vi "GUI TWM setup.vi"(0 "Common properties":T1={"Measurement status ref"=refnum, "TWM Status ref"=refnum, "Abort ref"=refnum, "Skip waiting ref"=refnum, "GNU Octave path"=path "C:/Program Files/GNU Octave/Octave-6.2.0/mingw64/bin", "TWM+QWTB path"=path "C:/Users/labina/Desktop/TWM-1.8.7.0-full/octprog", "lvlib path"=path "D:/martin/WAC/WACsw - github/control_software/Filter function meter/external libraries/GOLPI 0.7.3.1 source distribution LV 20.0 32 bit/lv_proc.dll", "TWM pipe"="\\\\.\\pipe\\TWM:server", "PJVS status ref"=refnum, "WAC path"=path ""}) -> (7 "Common properties out":T1={"Measurement status ref"=refnum, "TWM Status ref"=refnum, "Abort ref"=refnum, "Skip waiting ref"=refnum, "GNU Octave path"=path "C:/Program Files/GNU Octave/Octave-6.2.0/mingw64/bin", "TWM+QWTB path"=path "C:/Users/labina/Desktop/TWM-1.8.7.0-full/octprog", "lvlib path"=path "D:/martin/WAC/WACsw - github/control_software/Filter function meter/external libraries/GOLPI 0.7.3.1 source distribution LV 20.0 32 bit/lv_proc.dll", "TWM pipe"="\\\\.\\pipe\\TWM:server", "PJVS status ref"=refnum, "WAC path"=path ""})   [LabVIEW 2020]
doc: "GUI to set up connection to the sampling sotware TWM and to set up paths to calculation software GNU Octave."
uses:
  Utilities/Type definitions/Common properties.ctl
  <vilib>/Utility/error.llb/DialogType.ctl
  <vilib>/Utility/error.llb/Error Cluster From Error Code.vi
  <vilib>/ErrorRing/Error Ring.xnode
  external libraries/varilib/varilib.lvlib
  external libraries/TWM-1.8.7.0-client/TWM Client.lvlib
panel:
  in  "start octave":bool
  out "twm_qwtb_not_valid":string="not valid!"
  out "octave_not_valid":string="not valid!"
  in  "TWM+QWTB path":path=path "C:/Users/labina/Desktop/TWM-1.8.7.0-full/octprog"
  in  "GNU Octave path":path=path "C:/Program Files/GNU Octave/Octave-6.2.0/mingw64/bin"
  in  "TWM pipe":string="\\\\.\\pipe\\TWM:server"
  out "gui_elements":refnum<vi>[](array[refnum])
  out "Status":string
  in  "save_and_quit":bool
  in  "test TWM":bool
  in  "cancel":bool
  # "This software changes following properties\nin the TWM automatically before running \na measurement:\n1, Sampling rate (TWM->Setup Measurement)\n2, Samples count (TWM->Setup Measurement)\n3, Records count (TWM->Setup Measurement)\n4, Sub-records count (TWM->Setup Measurement)\n5, Trigger (mode, source, level, coupling\n                                     (TWM->Setup Measurment)\n6, Measurement name (TWM->Setup Measurement)\n7, Processing setup"
  # "You must set following in TWM\nby yourself:\n1, Octave/Matlab\n2, Digitizer"
  # "GNU Octave for calculation of results or recalculation of sampled data."
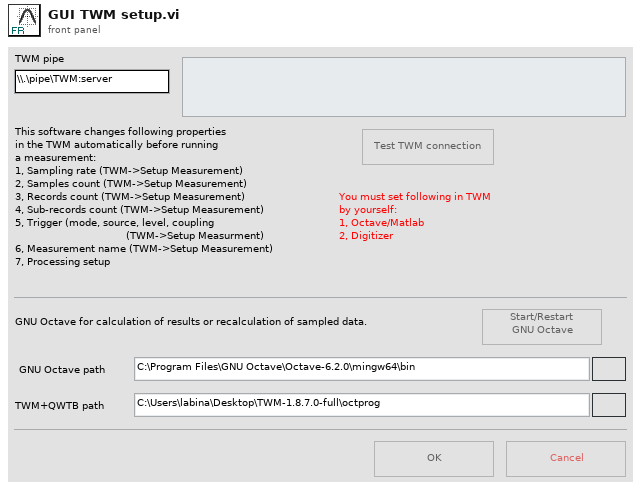
[diagram p1: front panel]
types:
  T1 = typedef "Common properties.ctl" = cluster{"Measurement status ref":refnum<vi>, "TWM Status ref":refnum<vi>, "Abort ref":refnum<vi>, "Skip waiting ref":refnum<vi>, "GNU Octave path":path, "TWM+QWTB path":path, "lvlib path":path, "TWM pipe":string, "PJVS status ref":refnum<vi>, "WAC path":path}
  T2 = typedef "DialogType.ctl" = u16
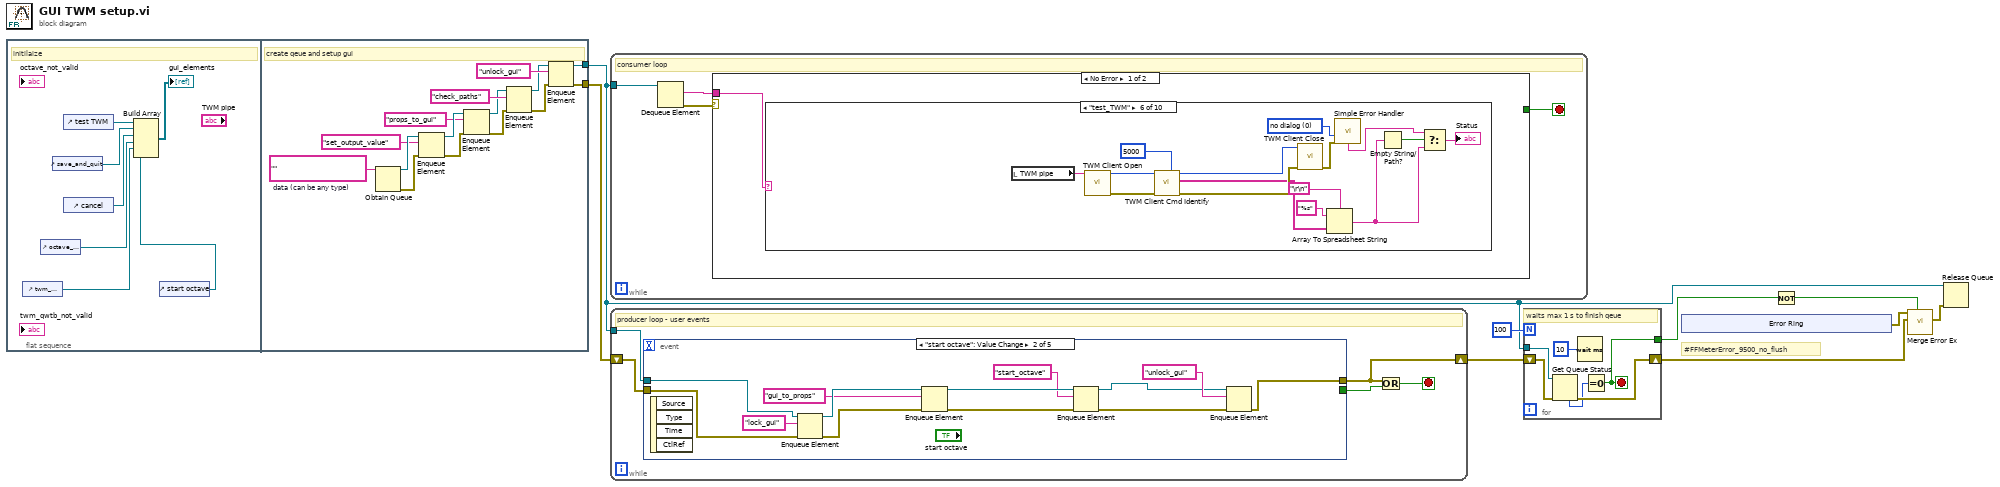
[diagram p0: block diagram]
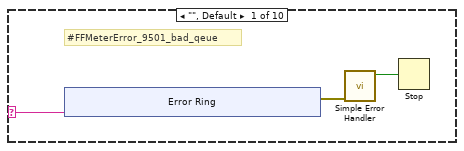
[diagram p2: hidden frame]
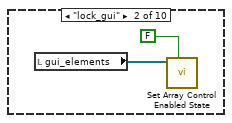
[diagram p3: hidden frame]
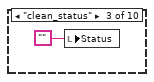
[diagram p4: hidden frame]
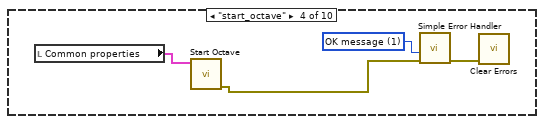
[diagram p5: hidden frame]
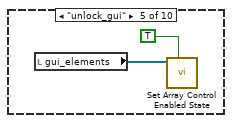
[diagram p6: hidden frame]
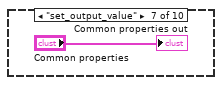
[diagram p7: hidden frame]
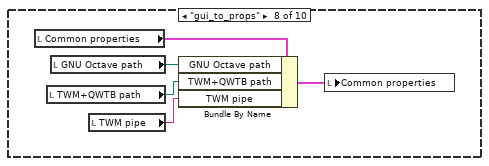
[diagram p8: hidden frame]
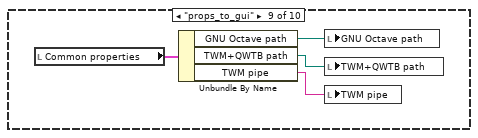
[diagram p9: hidden frame]
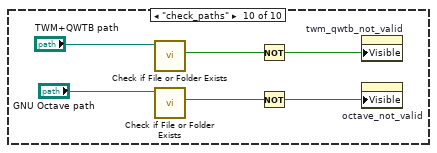
[diagram p10: hidden frame]
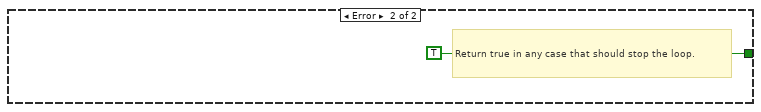
[diagram p11: hidden frame]
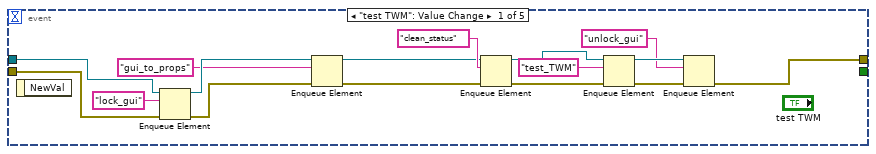
[diagram p12: hidden frame]
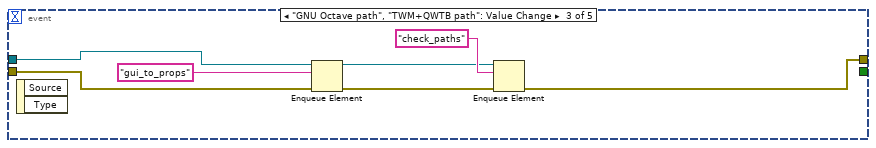
[diagram p13: hidden frame]
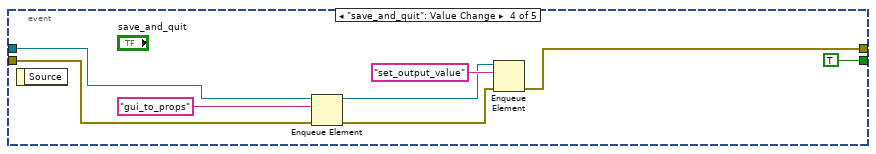
[diagram p14: hidden frame]
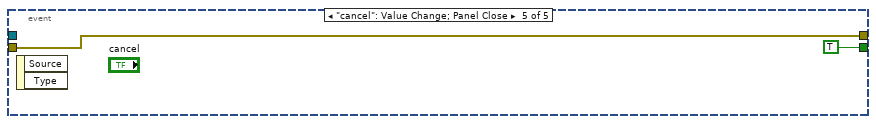
[diagram p15: hidden frame]
diagram:
  # "#FFMeterError_9500_no_flush"
  n1 = flat-sequence {
    tunnel: [w27] -> w2
    tunnel: [w25] -> w1
    frame #0 {
      # "initilaize"
      n2 = control-ref of="twm_qwtb_not_valid"() -> (w11:refnum<vi>)
      n3 = control-ref of="octave_not_valid"() -> (w12:refnum<vi>)
      n4 = control-ref of="save_and_quit"() -> (w15:refnum<vi>)
      n5 = control-ref of="test TWM"() -> (w16:refnum<vi>)
      n6 = control-ref of="cancel"() -> (w14:refnum<vi>)
      n7 = control-ref of="start octave"() -> (w10:refnum<vi>)
      n8 = Build Array(w16, w15, w14, w12, w11, w10) -> (→"gui_elements":refnum<vi>[])
    }
    frame #1 {
      w26 = ""  # data (can be any type)
      # "create qeue and setup gui"
      n9 = Obtain Queue(element data type=w26) -> (queue out=w30:refnum<queue>, error out=w31:errorcluster)  [unwired: 4 in, 1 out]
      n10 = Enqueue Element(queue=w30, element="set_output_value", error in (no error)=w31) -> (queue out=w18:refnum<queue>, error out=w21:errorcluster)  [unwired: 1 in, 1 out]
      n11 = Enqueue Element(queue=w18, element="props_to_gui", error in (no error)=w21) -> (queue out=w19:refnum<queue>, error out=w20:errorcluster)  [unwired: 1 in, 1 out]
      n12 = Enqueue Element(queue=w19, element="check_paths", error in (no error)=w20) -> (queue out=w23:refnum<queue>, error out=w24:errorcluster)  [unwired: 1 in, 1 out]
      n13 = Enqueue Element(queue=w23, element="unlock_gui", error in (no error)=w24) -> (queue out=w27:refnum<queue>, error out=w25:errorcluster)  [unwired: 1 in, 1 out]
    }
  }
  n14 = while {
    tunnel: w2 -> [w35]
    stop <- w32 stop-if-true
    # "consumer loop"
    n15 = Dequeue Element(queue=w35) -> (element=w33:string, error out=w34:errorcluster)  [unwired: 2 in, 2 out]
    n16 = case shown="No Error" w34 {
      tunnel: w33 -> [w36 _]
      tunnel: [_ TRUE] -> w32
      frame No Error {
        n17 = case shown="\"test_TWM\"" w36 {
          selector: w36 -> [w37 _ _ _ _ _ _ _ _ _]
          frame "", Default {
            # "#FFMeterError_9501_bad_qeue"
            n18 = xnode "Error Ring"("parameter 0"=w37) -> ("error out"=w39:errorcluster)
            n19 = call <vilib>:"Simple Error Handler.vi"("error in (no error)"=w39) -> ("error?"=w38:bool)  [unwired: 4 in, 4 out]
            n20 = Stop(stop? (T)=w38) -> ()
          }
          frame "lock_gui" {
            n21 = local read "gui_elements"() -> (w48:refnum<vi>[])
            n22 = call "Set Array Control Enabled State.vi"("enabled (T)"=FALSE, "reference array in"=w48) -> ()  [unwired: 8 in, 2 out]
          }
          frame "clean_status" {
            n23 = local write "Status"("") -> ()
          }
          frame "start_octave" {
            w52 = T2 1 items=["no dialog", "OK message", "continue or stop message", "OK message + warnings", "continue/stop + warnings"] ("type of dialog (OK msg:1)")
            n24 = local read "Common properties"() -> (w53:T1)
            n25 = call "Start Octave.vi"("Common properties"=w53) -> ("error out"=w51:errorcluster)  [unwired: 10 in]
            n26 = call <vilib>:"Simple Error Handler.vi"("type of dialog (OK msg:1)"=w52, "error in (no error)"=w51) -> ("error out"=w50:errorcluster)  [unwired: 3 in, 4 out]
            n27 = call <vilib>:"Clear Errors.vi"("error in (no error)"=w50) -> ()  [unwired: 5 in, 2 out]
          }
          frame "unlock_gui" {
            n28 = local read "gui_elements"() -> (w55:refnum<vi>[])
            n29 = call "Set Array Control Enabled State.vi"("enabled (T)"=TRUE, "reference array in"=w55) -> ()  [unwired: 8 in, 2 out]
          }
          frame "test_TWM" {
            w61 = T2 0 items=["no dialog", "OK message", "continue or stop message", "OK message + warnings", "continue/stop + warnings"] ("type of dialog (OK msg:1)")
            n30 = local read "TWM pipe"() -> (w57:string)
            n31 = call "TWM Client Open.vi"("pipe name"=w57) -> ("error out"=w69:errorcluster, "handle out"=w68:i32)  [unwired: 9 in]
            n32 = call "TWM Client Cmd Identify.vi"("timeout [ms]"=5000, "error in"=w69, "handle"=w68) -> ("error out"=w70:errorcluster, "channel idns"=w65:string[], "handle out"=w67:i32)  [unwired: 5 in, 1 out]
            n33 = call "TWM Client Close.vi"("error in"=w70, "handle in"=w67) -> ("error out"=w62:errorcluster)  [unwired: 9 in]
            n34 = Array To Spreadsheet String(delimiter (Tab)="\r\n", array=w65, 3:"%s" ("format string")) -> (spreadsheet string=w58:string)
            n35 = call <vilib>:"Simple Error Handler.vi"("type of dialog (OK msg:1)"=w61, "error in (no error)"=w62) -> ("message"=w59:string)  [unwired: 3 in, 4 out]
            n36 = Empty String/Path?(string/path=w58) -> (empty?=w60:bool)
            n37 = Select(t=w59, s=w60, f=w58) -> (s? t:f=→"Status":string)
          }
          frame "set_output_value" {
            "Common properties out" <- "Common properties"
          }
          frame "gui_to_props" {
            n38 = local read "Common properties"() -> (w76:T1)
            n39 = local read "TWM+QWTB path"() -> (w73:path)
            n40 = local read "GNU Octave path"() -> (w74:path)
            n41 = local read "TWM pipe"() -> (w72:string)
            n42 = Bundle By Name(cluster=w76, "GNU Octave path"=w74, "TWM+QWTB path"=w73, "TWM pipe"=w72) -> (w75:T1)
            n43 = local write "Common properties"(w75) -> ()
          }
          frame "props_to_gui" {
            n44 = local read "Common properties"() -> (w80:T1)
            n45 = Unbundle By Name(w80) -> ("GNU Octave path"=w79:path, "TWM+QWTB path"=w78:path, "TWM pipe"=w77:string)
            n46 = local write "GNU Octave path"(w79) -> ()
            n47 = local write "TWM+QWTB path"(w78) -> ()
            n48 = local write "TWM pipe"(w77) -> ()
          }
          frame "check_paths" {
            n49 = call <vilib>:"Check if File or Folder Exists.vi"("path"="TWM+QWTB path") -> ("file or folder exists?"=w82:bool)  [unwired: 8 in, 2 out]
            n50 = call <vilib>:"Check if File or Folder Exists.vi"("path"="GNU Octave path") -> ("file or folder exists?"=w85:bool)  [unwired: 8 in, 2 out]
            n51 = Not(x=w82) -> (.not. x?=w81:bool)
            n52 = Not(x=w85) -> (.not. x?=w84:bool)
            n53 = property on="twm_qwtb_not_valid" class="Str"("Visible"=w81) -> ()  [unwired: 2 in, 2 out]
            n54 = property on="octave_not_valid" class="Str"("Visible"=w84) -> ()  [unwired: 2 in, 2 out]
          }
        }
      }
      frame Error {
        # "Return true in any case that should stop the loop."
      }
    }
  }
  n55 = while {
    shift-right: [w88] -> w5
    shift-left: w1 -> [w91]
    tunnel: w2 -> [w92]
    stop <- w89 stop-if-true
    # "producer loop - user events"
    n56 = event shown="[1] \"start octave\": Value Change" {
      selector: _ -> [_ _ _ _ _]
      dyn-events: _ -> [_ _ _ _ _]
      timeout: _ -> [_ _ _ _ _]
      tunnel: w92 -> [w102 w111 w127 w134 _]
      tunnel: w91 -> [w103 w113 w126 w133 w138]
      tunnel: [w106 w112 w122 w129 w138] -> w88
      tunnel: [_ _ _ TRUE ("cancel") TRUE ("cancel")] -> w90
      event "test TWM": Value Change {
        n57 = event-data() -> ()  [unwired: 1 in, 1 out]
        n58 = Enqueue Element(queue=w102, element="lock_gui", error in (no error)=w103) -> (queue out=w99:refnum<queue>, error out=w100:errorcluster)  [unwired: 1 in, 1 out]
        n59 = Enqueue Element(queue=w99, element="gui_to_props", error in (no error)=w100) -> (queue out=w95:refnum<queue>, error out=w96:errorcluster)  [unwired: 1 in, 1 out]
        n60 = Enqueue Element(queue=w95, element="clean_status", error in (no error)=w96) -> (queue out=w93:refnum<queue>, error out=w94:errorcluster)  [unwired: 1 in, 1 out]
        n61 = Enqueue Element(queue=w93, element="test_TWM", error in (no error)=w94) -> (queue out=w105:refnum<queue>, error out=w107:errorcluster)  [unwired: 1 in, 1 out]
        n62 = Enqueue Element(queue=w105, element="unlock_gui", error in (no error)=w107) -> (error out=w106:errorcluster)  [unwired: 1 in, 2 out]
      }
      event "start octave": Value Change {
        n63 = event-data() -> ()  [unwired: 1 in, 4 out]
        n64 = Enqueue Element(queue=w111, element="lock_gui", error in (no error)=w113) -> (queue out=w120:refnum<queue>, error out=w121:errorcluster)  [unwired: 1 in, 1 out]
        n65 = Enqueue Element(queue=w120, element="gui_to_props", error in (no error)=w121) -> (queue out=w118:refnum<queue>, error out=w119:errorcluster)  [unwired: 1 in, 1 out]
        n66 = Enqueue Element(queue=w118, element="start_octave", error in (no error)=w119) -> (queue out=w110:refnum<queue>, error out=w109:errorcluster)  [unwired: 1 in, 1 out]
        n67 = Enqueue Element(queue=w110, element="unlock_gui", error in (no error)=w109) -> (error out=w112:errorcluster)  [unwired: 1 in, 2 out]
      }
      event "GNU Octave path", "TWM+QWTB path": Value Change {
        n68 = event-data() -> ()  [unwired: 1 in, 2 out]
        n69 = Enqueue Element(queue=w127, element="gui_to_props", error in (no error)=w126) -> (queue out=w123:refnum<queue>, error out=w124:errorcluster)  [unwired: 1 in, 1 out]
        n70 = Enqueue Element(queue=w123, element="check_paths", error in (no error)=w124) -> (error out=w122:errorcluster)  [unwired: 1 in, 2 out]
      }
      event "save_and_quit": Value Change {
        n71 = event-data() -> ()  [unwired: 1 in, 1 out]
        n72 = Enqueue Element(queue=w134, element="gui_to_props", error in (no error)=w133) -> (queue out=w130:refnum<queue>, error out=w131:errorcluster)  [unwired: 1 in, 1 out]
        n73 = Enqueue Element(queue=w130, element="set_output_value", error in (no error)=w131) -> (error out=w129:errorcluster)  [unwired: 1 in, 2 out]
      }
      event "cancel": Value Change; Panel Close {
        n74 = event-data() -> ()  [unwired: 1 in, 2 out]
      }
    }
    n75 = Or(x=w88, y=w90) -> (x .or. y?=w89:bool)
  }
  n76 = for {
    N: 100 -> [_]
    tunnel: w2 -> [w144]
    shift-right: [w142] -> w6
    shift-left: w5 -> [w143]
    tunnel: [w139] -> w3
    stop <- w139 stop-if-true
    # "waits max 1 s to finish qeue"
    n77 = Get Queue Status(queue=w144, error in (no error)=w143) -> (error out=w142:errorcluster, # elements in queue=w140:i32)  [unwired: 1 in, 6 out]
    n78 = Wait (ms)(milliseconds to wait=u32 10) -> ()  [unwired: 1 out]
    n79 = Equal To 0?(x=w140) -> (x = 0?=w139:bool)
  }
  n80 = xnode "Error Ring"() -> ("error out"=w7:errorcluster)
  n81 = Not(x=w3) -> (.not. x?=w8:bool)
  n82 = call "Merge Error Ex.vi"("Is error? (False)"=w8, "main error in (no error)"=w6, "second error in"=w7) -> ("error out"=w4:errorcluster)  [unwired: 8 in]
  n83 = Release Queue(queue=w2, error in (no error)=w4) -> ()  [unwired: 1 in, 3 out]
